vi "Build Pose Target Array.vi"(7 "Current Pose":T1, 9 "Pose Position Target":T1, 10 "Pose Name Target":T2, 11 "Pose Config":T3[](array[typedef])) -> (2 "Valid Value Out":bool, 3 "Pose Targets Out":T1[](array[typedef]))   [LabVIEW 2020, in "MotionMaster_SubCMD.lvlib"]
uses:
  MotionMaster_SubCMD.lvlib
  Shared Code/TypeDefs/Cluster_Pose Positions.ctl
  ENUM_Pose List.ctl
  Shared Code/TypeDefs/Cluster_Pose Name and  Data.ctl
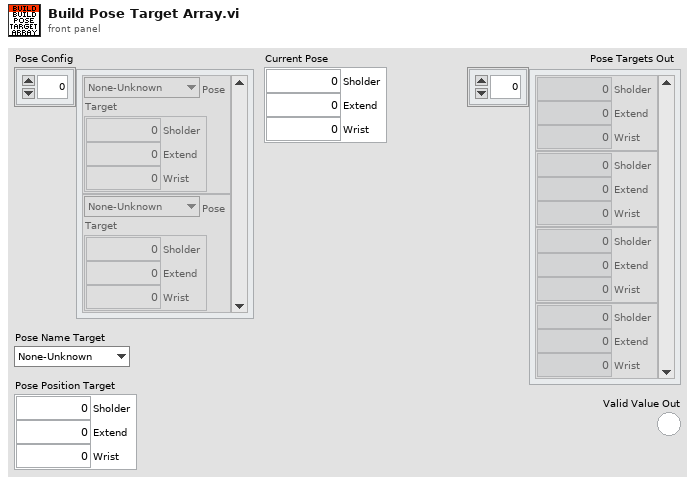
[diagram p1: front panel]
types:
  T1 = typedef "Cluster_Pose Positions.ctl" = cluster{"Sholder":i32, "Extend":i32, "Wrist":i32}
  T2 = typedef "MotionMaster_SubCMD.lvlib/ENUM_Pose List.ctl" = enum16{"None-Unknown", "Parked", "Intaking", "Med Goal", "High Goal"}
  T3 = typedef "Cluster_Pose Name and  Data.ctl" = cluster{"Pose":T2, "Target":T1}
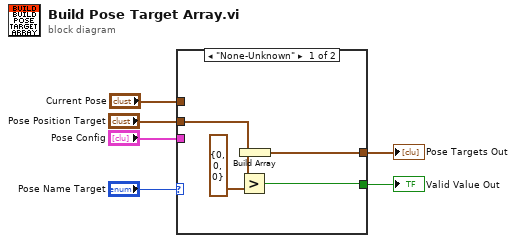
[diagram p0: block diagram]
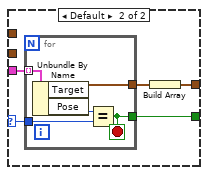
[diagram p2: hidden frame]
diagram:
  n1 = case shown="\"None-Unknown\"" "Pose Name Target" {
    selector: "Pose Name Target" -> [_ w14]
    tunnel: "Pose Config" -> [_ w15]
    tunnel: "Pose Position Target" -> [w9 _]
    tunnel: [w10 w11] -> w3
    tunnel: [w7 w13] -> w2
    tunnel: "Current Pose" -> [_ _]
    frame "None-Unknown" {
      n2 = Greater?(x=w9, y=T1 {"Sholder"=0, "Extend"=0, "Wrist"=0}) -> (0:w7:bool)
      n3 = Build Array(w9) -> (w10:T1[])
    }
    frame Default {
      n4 = for {
        tunnel: w15 -> [w20] mode=indexing
        tunnel: w14 -> [w19]
        tunnel: [w17] -> w13
        tunnel: [w16] -> w12
        stop <- w17 stop-if-true
        n5 = Unbundle By Name(w20) -> ("Target"=w16:T1, "Pose"=w18:T2)
        n6 = Equal?(x=w18, y=w19) -> (x = y?=w17:bool)
      }
      n7 = Build Array(w12) -> (w11:T1[])
    }
  }
  "Pose Targets Out" <- w3
  "Valid Value Out" <- w2
